vi "MIDTERM EXAM.vi"(0 "Delay Time (s)":dbl=1.0) -> (1 "Number of Equations Proven True":dbl, 2 "Array Containing\nTrue Equations":i32[][](array[numeric]))   [LabVIEW 2010]
doc: "VI that outputs an erray of equations one per specified second(s) along with the number of equations proven true."
panel:
  # "D O G C A T"
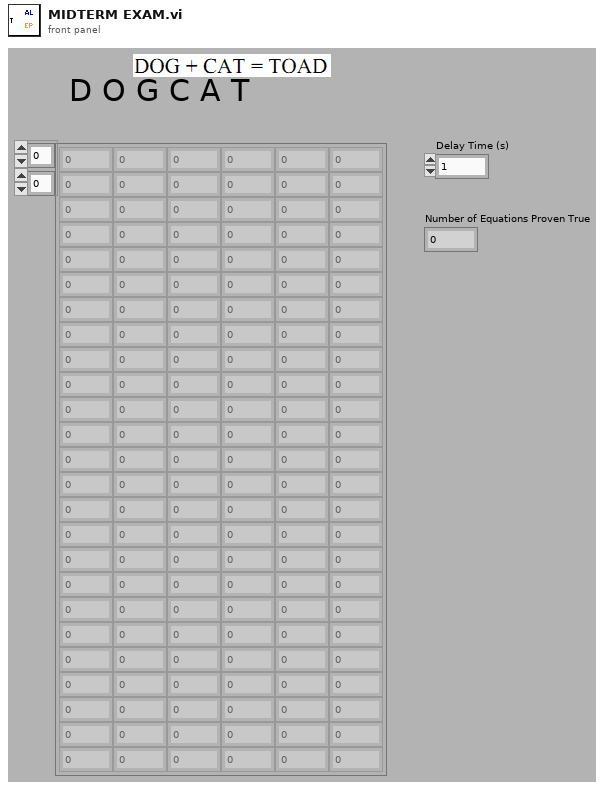
[diagram p1: front panel]
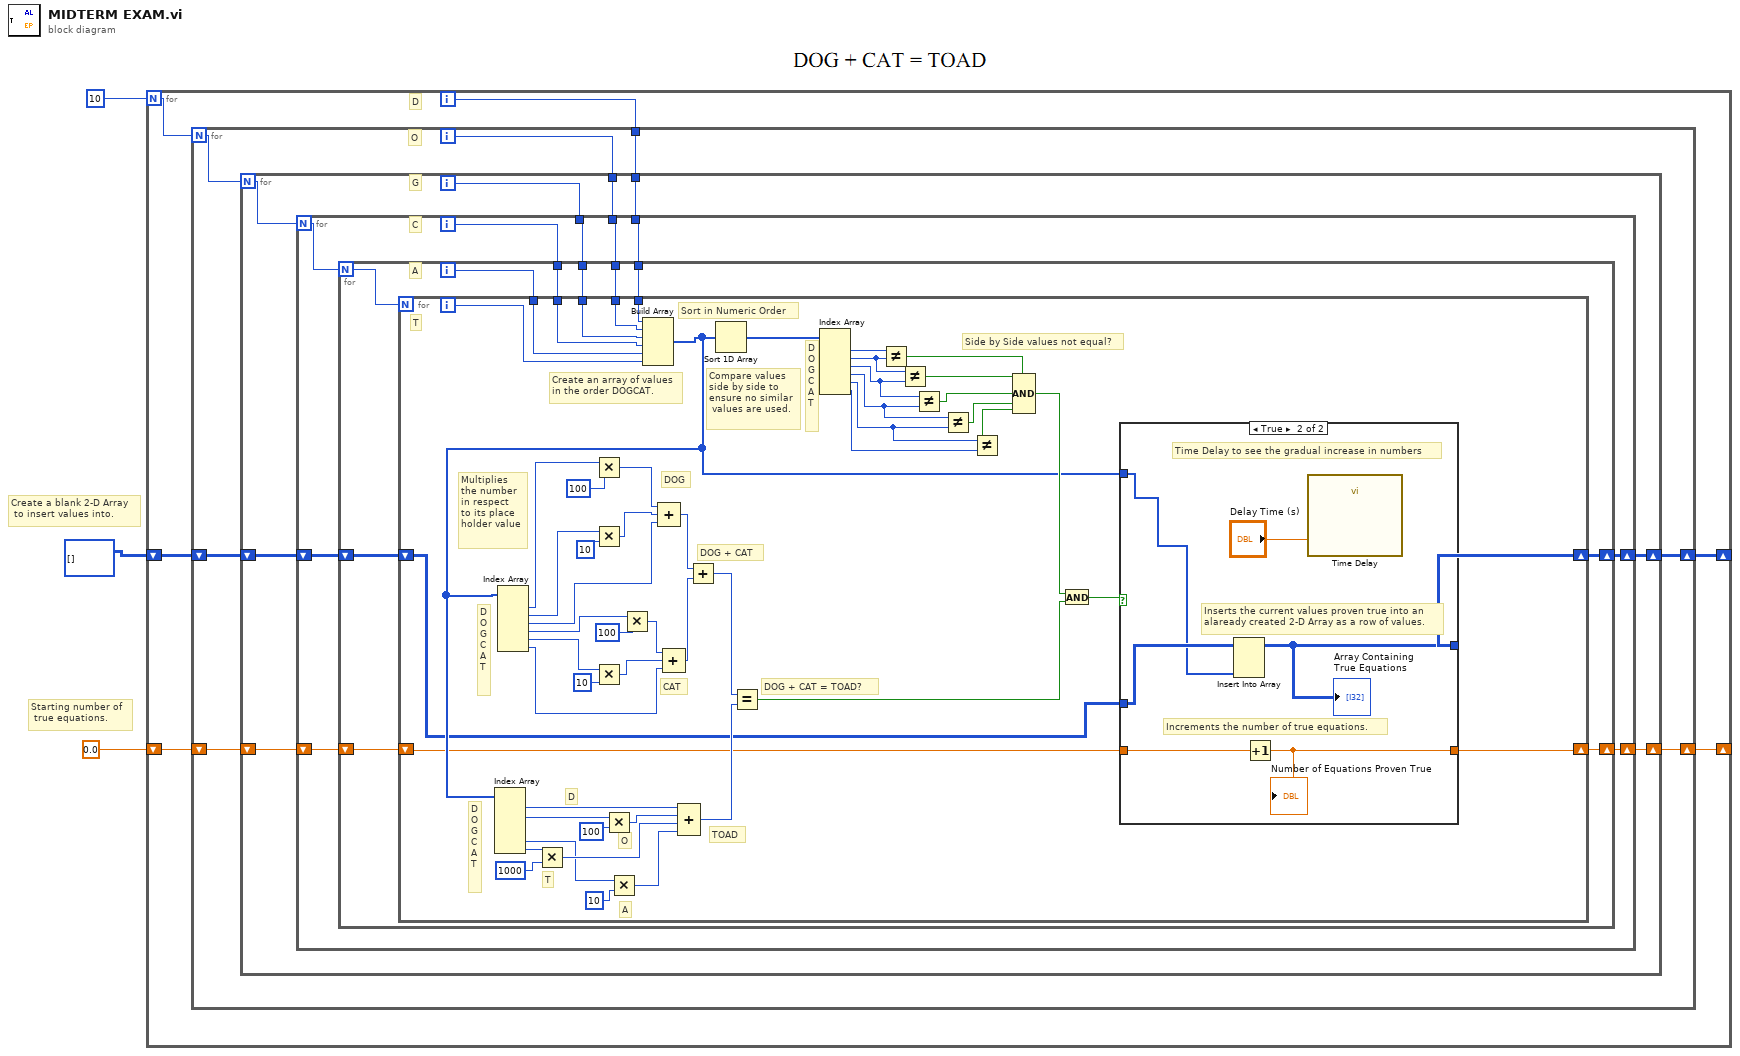
[diagram p0: block diagram]
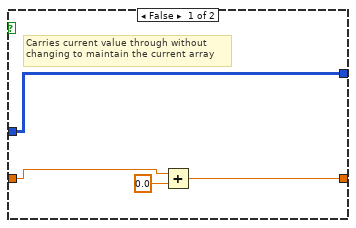
[diagram p2: hidden frame]
diagram:
  # "Starting number of\n true equations."
  # "Create a blank 2-D Array\n to insert values into."
  n1 = for {
    N: 10 -> [w9]
    shift-right: [w6] -> _
    shift-left: 0.0 -> [w7]
    shift-right: [w4] -> _
    shift-left: i32[][] [] -> [w5]
    i -> [w8]
    # "D"
    n2 = for {
      N: w9 -> [w16]
      tunnel: w8 -> [w15]
      shift-right: [w12] -> w6
      shift-left: w7 -> [w13]
      shift-right: [w10] -> w4
      shift-left: w5 -> [w11]
      i -> [w14]
      # "O"
      n3 = for {
        N: w16 -> [w24]
        tunnel: w15 -> [w23]
        tunnel: w14 -> [w22]
        shift-right: [w19] -> w12
        shift-left: w13 -> [w20]
        shift-right: [w17] -> w10
        shift-left: w11 -> [w18]
        i -> [w21]
        # "G"
        n4 = for {
          N: w24 -> [w33]
          tunnel: w23 -> [w32]
          tunnel: w22 -> [w31]
          tunnel: w21 -> [w30]
          shift-right: [w27] -> w19
          shift-left: w20 -> [w28]
          shift-right: [w25] -> w17
          shift-left: w18 -> [w26]
          i -> [w29]
          # "C"
          n5 = for {
            N: w33 -> [w43]
            tunnel: w32 -> [w42]
            tunnel: w31 -> [w41]
            tunnel: w30 -> [w40]
            tunnel: w29 -> [w39]
            shift-right: [w36] -> w27
            shift-left: w28 -> [w37]
            shift-right: [w34] -> w25
            shift-left: w26 -> [w35]
            i -> [w38]
            # "A"
            n6 = for {
              N: w43 -> [_]
              tunnel: w42 -> [w97]
              tunnel: w41 -> [w96]
              tunnel: w40 -> [w95]
              tunnel: w39 -> [w94]
              tunnel: w38 -> [w82]
              shift-right: [w46] -> w36
              shift-left: w37 -> [w47]
              shift-right: [w44] -> w34
              shift-left: w35 -> [w45]
              i -> [w81]
              # "T"
              # "Create an array of values\nin the order DOGCAT."
              # "Sort in Numeric Order"
              # "Multiplies \nthe number\nin respect\nto its place\nholder value"
              # "Side by Side values not equal?"
              # "DOG + CAT = TOAD?"
              # "TOAD"
              # "D\nO\nG\nC\nA\nT"
              # "D\nO\nG\nC\nA\nT"
              # "D\nO\nG\nC\nA\nT"
              # "D"
              # "A"
              # "O"
              # "T"
              # "DOG + CAT"
              # "CAT"
              # "DOG"
              # "Compare values\nside by side to \nensure no similar\n values are used."
              n7 = Build Array(w97, w96, w95, w94, w82, w81) -> (w48:i32[])
              n8 = Index Array ("DOGCAT")(array=w48) -> (element #1=w74:i32, element #2=w70:i32, element #5=w72:i32, element #6=w68:i32)  [unwired: 6 in, 2 out]
              n9 = Index Array ("DOGCAT")(array=w48) -> (element #1=w54:i32, element #2=w55:i32, element #3=w62:i32, element #4=w58:i32, element #5=w56:i32, element #6=w63:i32)  [unwired: 6 in]
              n10 = Multiply(x=w68, y=1000) -> (x*y=w76:i32)
              n11 = Multiply(x=w54, y=100) -> (x*y=w52:i32)
              n12 = Multiply(x=w55, y=10) -> (x*y=w61:i32)
              n13 = Multiply(x=w56, y=10) -> (x*y=w64:i32)
              n14 = Multiply(x=w70, y=100) -> (x*y=w75:i32)
              n15 = Multiply(x=w72, y=10) -> (x*y=w77:i32)
              n16 = Multiply(x=w58, y=100) -> (x*y=w65:i32)
              n17 = Compound Arithmetic op=ADD(w52, w61, w62) -> (w66:i32)
              n18 = Compound Arithmetic op=ADD(w65, w64, w63) -> (w67:i32)
              n19 = Compound Arithmetic op=ADD(w74, w75, w76, w77) -> (w79:i32)
              n20 = Add(x=w66, y=w67) -> (x+y=w78:i32)
              n21 = Sort 1D Array(array=w48) -> (sorted array=w80:i32[])
              n22 = Equal?(x=w78, y=w79) -> (x = y?=w50:bool)
              n23 = Index Array(array=w80) -> (element #1=w93:i32, element #2=w92:i32, element #3=w91:i32, element #4=w90:i32, element #5=w89:i32, element #6=w88:i32)  [unwired: 6 in]
              n24 = Not Equal?(x=w93, y=w92) -> (x != y?=w87:bool)
              n25 = Not Equal?(x=w92, y=w91) -> (x != y?=w86:bool)
              n26 = Not Equal?(x=w91, y=w90) -> (x != y?=w85:bool)
              n27 = Not Equal?(x=w90, y=w89) -> (x != y?=w84:bool)
              n28 = Not Equal?(x=w89, y=w88) -> (x != y?=w83:bool)
              n29 = Compound Arithmetic op=AND(w87, w86, w85, w84, w83) -> (w51:bool)
              n30 = And(x=w51, y=w50) -> (x .and. y?=w49:bool)
              n31 = case shown="True" w49 {
                tunnel: w48 -> [_ w105]
                tunnel: [w99 w102] -> w46
                tunnel: w47 -> [w100 w104]
                tunnel: w45 -> [w98 w106]
                tunnel: [w98 w103] -> w44
                frame False {
                  # "Carries current value through without\nchanging to maintain the current array"
                  n32 = Add(x=w100, y=0.0) -> (x+y=w99:dbl)
                }
                frame True {
                  # "Time Delay to see the gradual increase in numbers"
                  # "Increments the number of true equations."
                  # "Inserts the current values proven true into an\nalaready created 2-D Array as a row of values."
                  n33 = Insert Into Array(array=w106, new element=w105) -> (w103:i32[][])  [unwired: 2 in]
                  "Array Containing\nTrue Equations" <- w103
                  n34 = Increment(x=w104) -> (x+1=w102:dbl)
                  "Number of Equations Proven True" <- w102
                  n35 = call "Time Delay"("Delay Time (s)"="Delay Time (s)") -> ()  [unwired: 10 in, 1 out]
                }
              }
            }
          }
        }
      }
    }
  }
